vi "_CSMOFGV.vi"(6 "Operation":T3=enum."Get By Name", 7 "Allowed Messages(Empty for all)":string[](array[string]), 8 "Error in":errorcluster caption="Error in (no error)", 10 "Reference":string, 11 "Name(\"\" to use uuid) in":string) -> (0 "Error out":errorcluster, 1 "Boolean":bool, 3 "Array":T1[](array[typedef]))   [LabVIEW 2020, in "Communicable State Machine.lvlib"]
uses:
  Communicable State Machine.lvlib
  _CSMOFGVOPER.ctl
  _CSMObj.ctl
  Priority Queue.lvclass
  _CSM_MODE.ctl
  _CSMObj-Data.ctl
  _CSM Status Change Event Data.ctl
  _CSMObj-ModeData.ctl
  Def-CSMOMgr.ctl
  Priority Queue.lvclass/Priority Queue.ctl
  global-CSMQ FGV Change Flag.vi
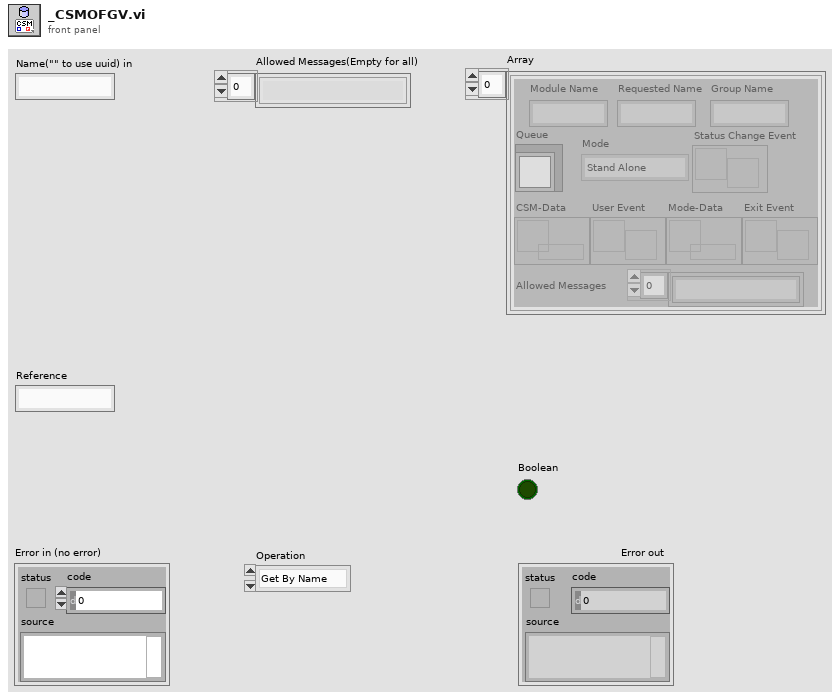
[diagram p1: front panel]
types:
  T1 = typedef "Communicable State Machine.lvlib/_CSMObj.ctl" = cluster{"Requested Name":string, "Module Name":string, "Mode":T2, "Queue":refnum<class "Priority Queue.lvclass">, "CSM-Data":refnum<data-value>, "User Event":refnum<user-event>, "Status Change Event":refnum<user-event>, "Allowed Messages":string[], "Mode-Data":refnum<data-value>, "Group Name":string, "Exit Event":refnum<user-event>}
  T2 = typedef "Communicable State Machine.lvlib/_CSM_MODE.ctl" = enum16{"Not Exist", "Stand Alone", "CSM", "Worker Agent", "Worker", "Chain", "Chain Node"}
  T3 = typedef "Communicable State Machine.lvlib/_CSMOFGVOPER.ctl" = enum16{"Create If not Exist", "Get By Name", "List", "Check If Name Exists", "Release", "Module Status", "Create Status Event Handler", "Destroy Status Event Handler"}
  T4 = typedef "Communicable State Machine.lvlib/Def-CSMOMgr.ctl" = variant
  T5 = typedef "Communicable State Machine.lvlib/_CSMObj-ModeData.ctl" = cluster{"Share Count":i32, "Messages of Chain Nodes":cluster{"Module Name":string, "Allowed Messages":string[]}[], "Chain Message Mapping Map":variant}
  T6 = cluster{"Module Name":string, "Allowed Messages":string[]}[]
  T7 = cluster{"Module Name":string, "Allowed Messages":string[]}
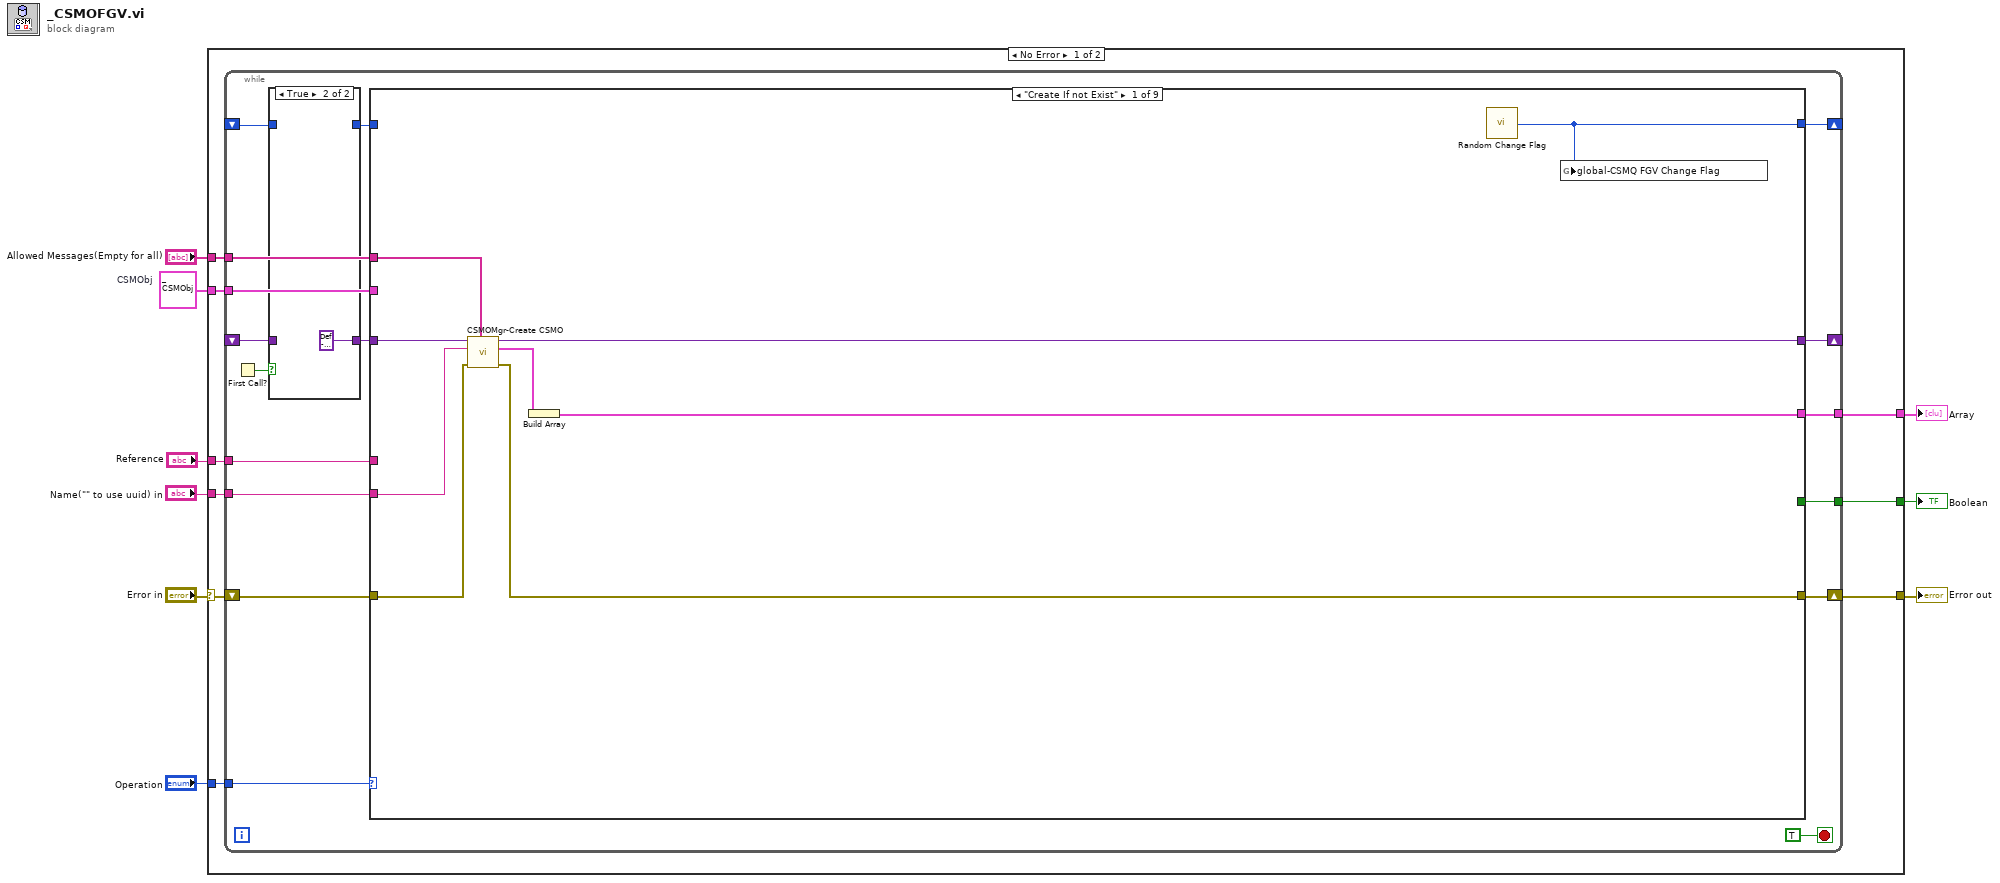
[diagram p0: block diagram]
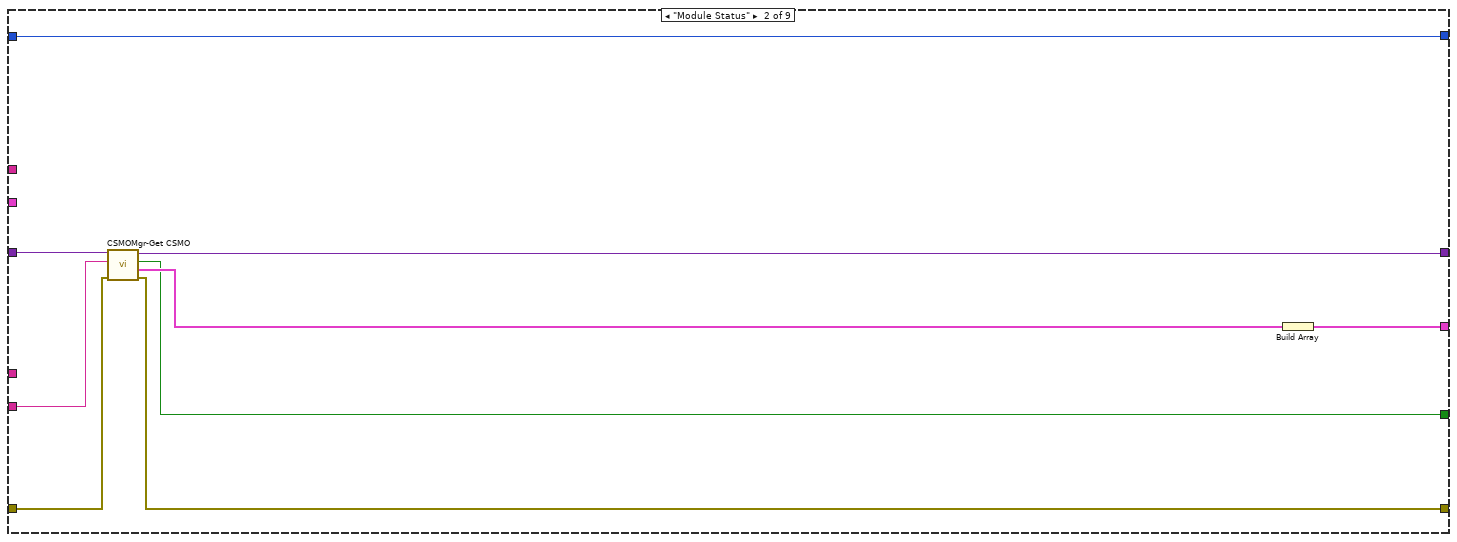
[diagram p3: hidden frame]
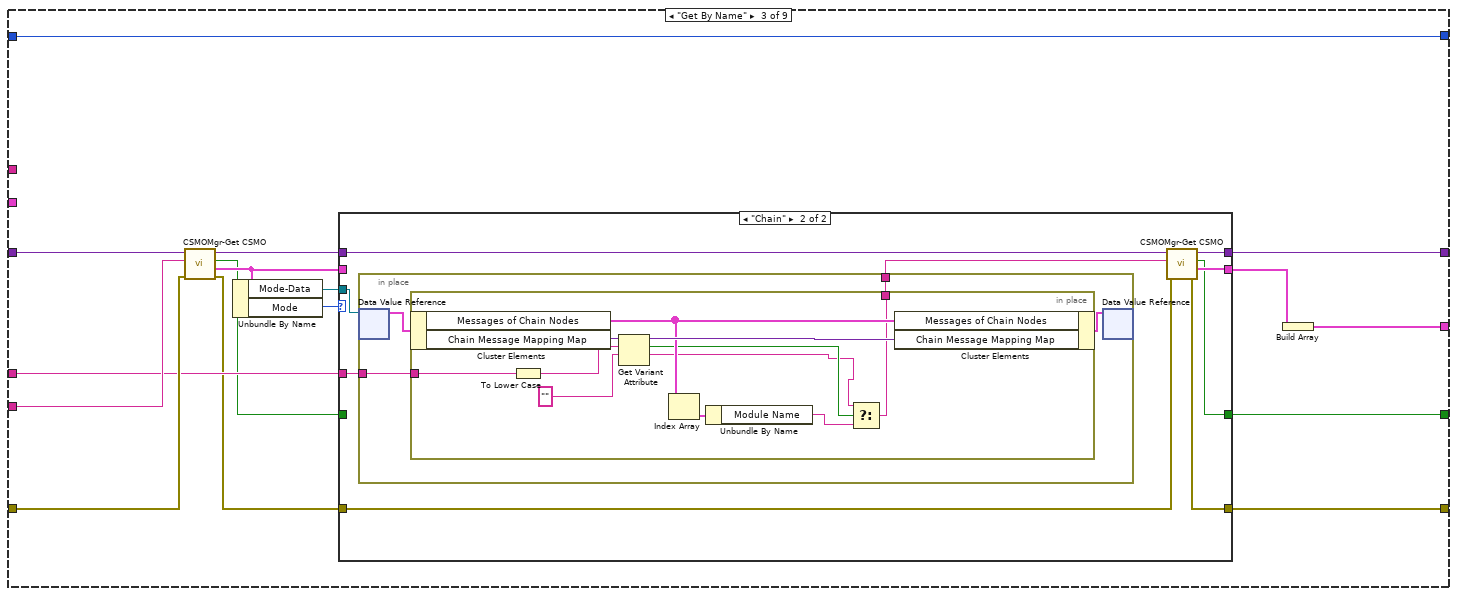
[diagram p4: hidden frame]
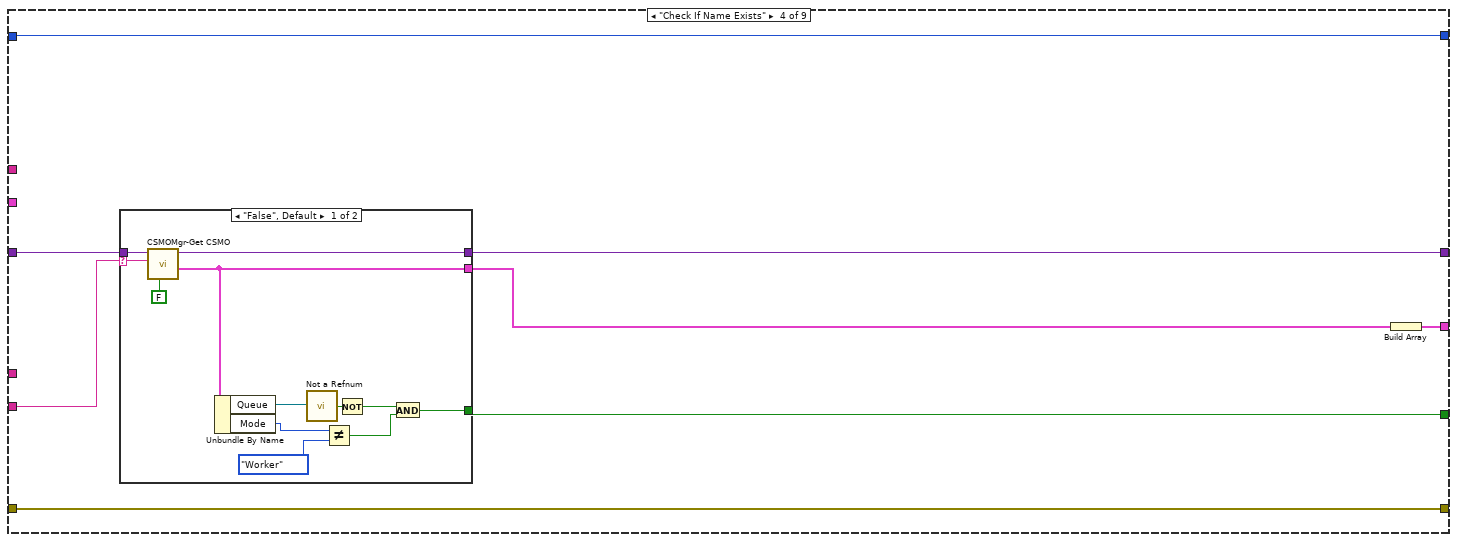
[diagram p6: hidden frame]
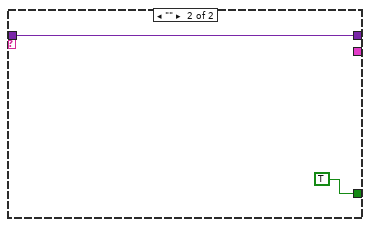
[diagram p7: hidden frame]
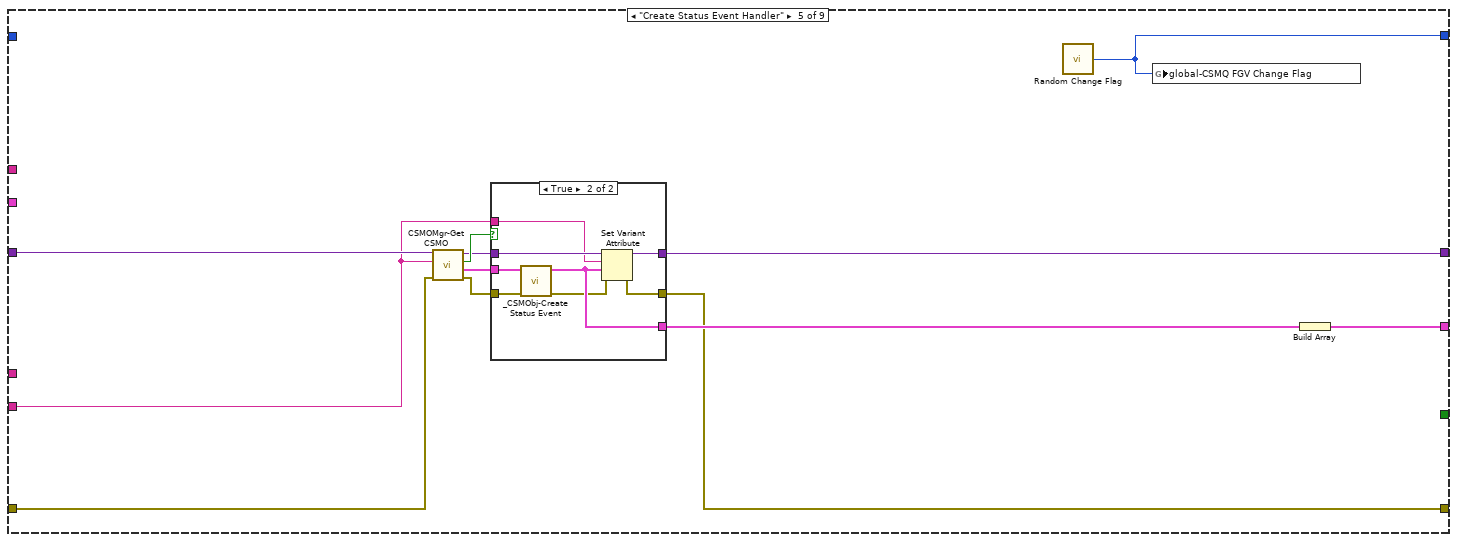
[diagram p8: hidden frame]
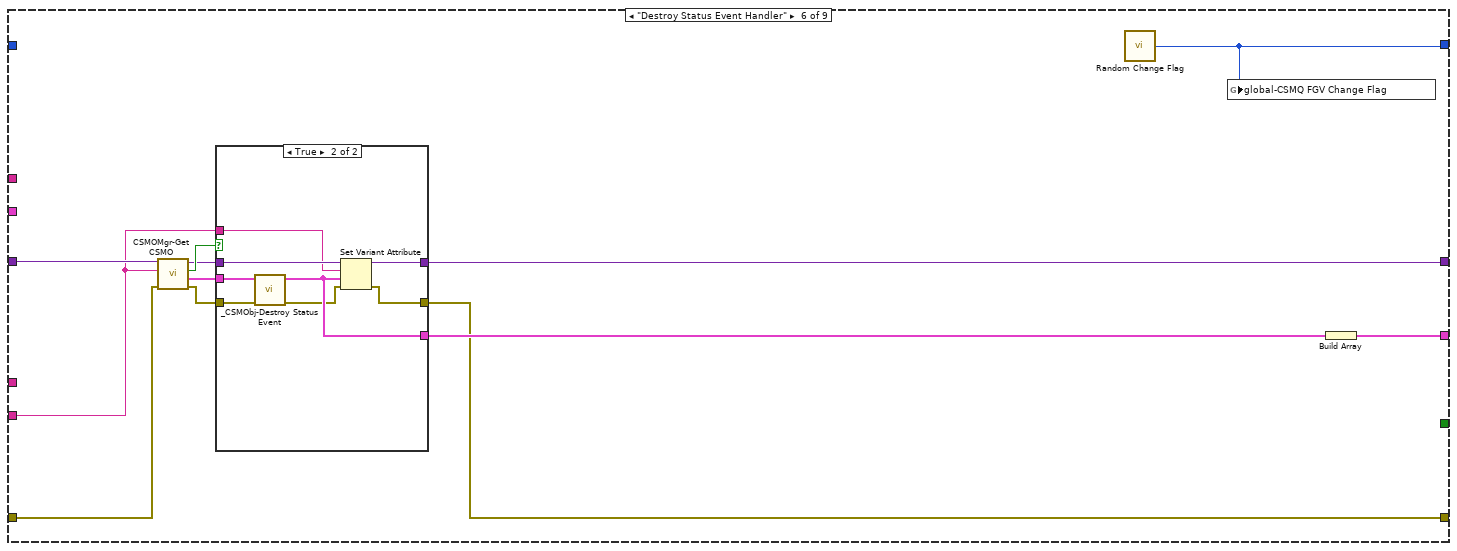
[diagram p10: hidden frame]
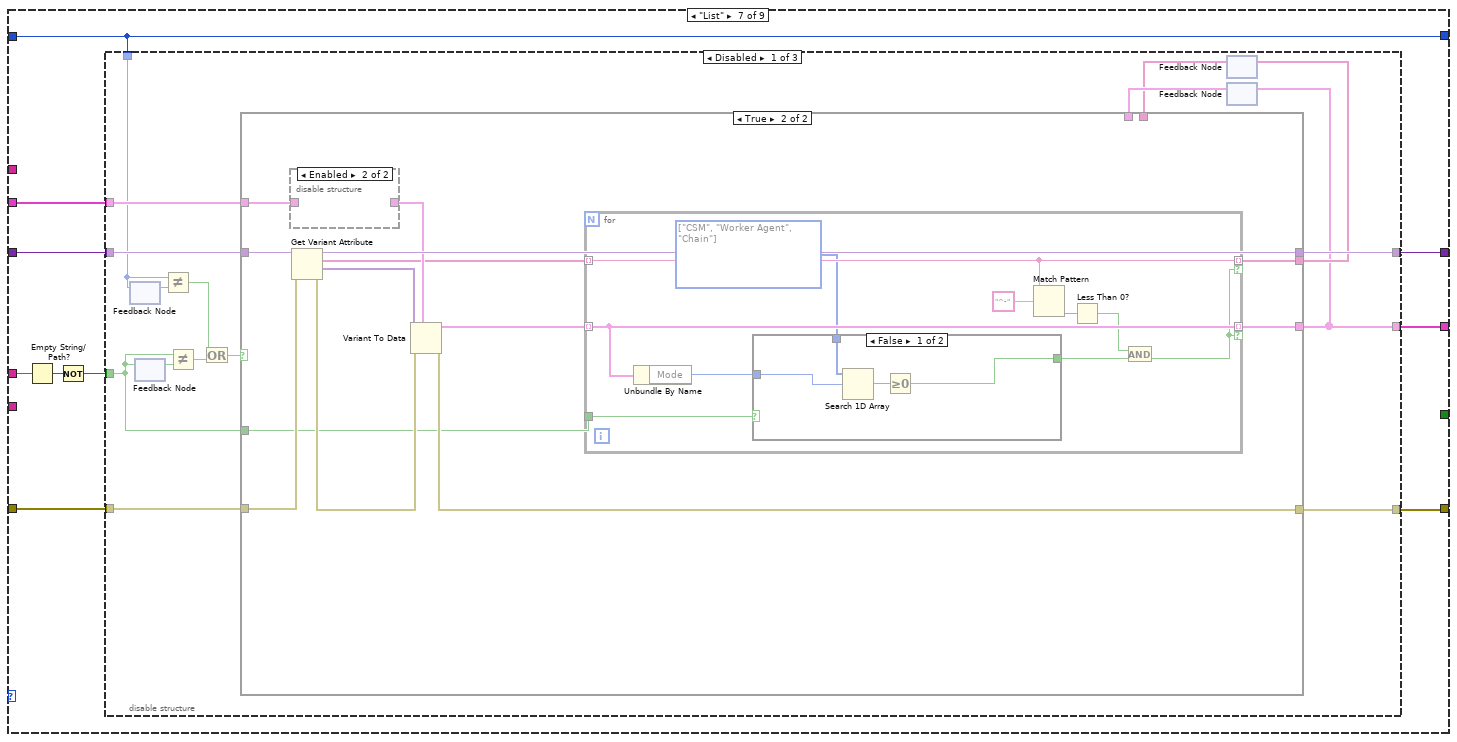
[diagram p12: hidden frame]
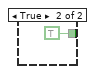
[diagram p14: hidden frame]
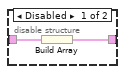
[diagram p15: hidden frame]
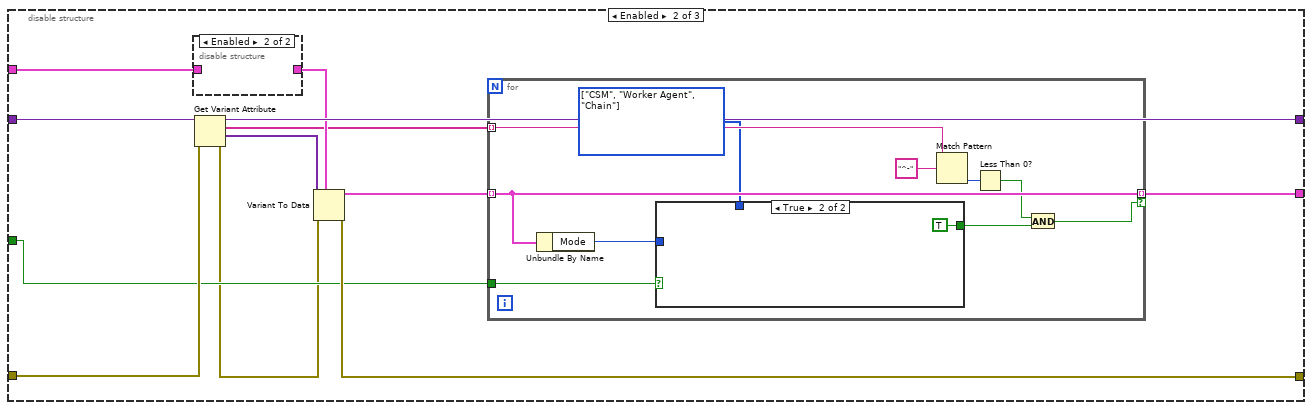
[diagram p16: hidden frame]
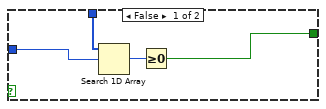
[diagram p17: hidden frame]
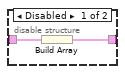
[diagram p18: hidden frame]
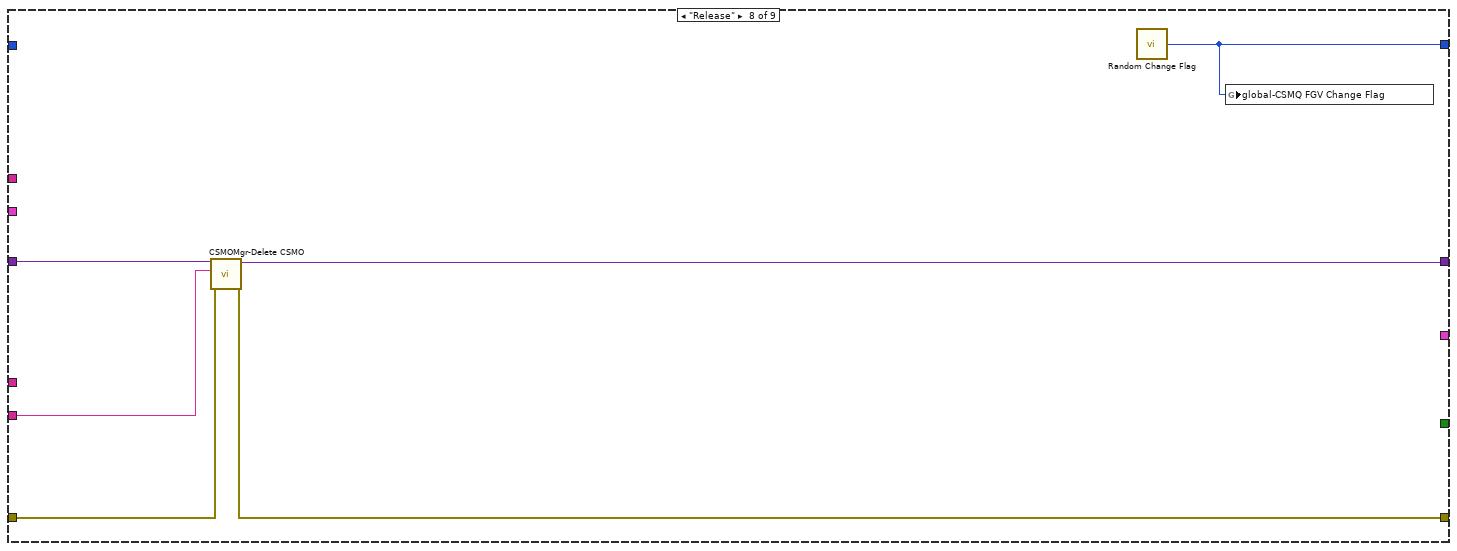
[diagram p20: hidden frame]
diagram:
  w5 = T1 {"Requested Name"="", "Module Name"="", "Mode"=enum."Stand Alone", "Queue"=refnum, "CSM-Data"=refnum, "User Event"=refnum, "Status Change Event"=refnum, "Allowed Messages"=[], "Mode-Data"=refnum, "Group Name"="", "Exit Event"=refnum}  # CSMObj
  n1 = case shown="No Error" "Error in" {
    selector: "Error in" -> [w16 w267]
    tunnel: "Operation" -> [w18 _]
    tunnel: "Name(\"\" to use uuid) in" -> [w17 _]
    tunnel: [w15 w267] -> w6
    tunnel: w5 -> [w14 _]
    tunnel: [w13 _] -> w4
    tunnel: [w12 _] -> w3
    tunnel: "Allowed Messages(Empty for all)" -> [w11 _]
    tunnel: "Reference" -> [w10 _]
    frame No Error {
      n2 = while {
        tunnel: w18 -> [w34]
        tunnel: w17 -> [w33]
        tunnel: [w32] -> w13
        shift-right: [w28] -> _
        shift-left: _ -> [w30]
        shift-right: [w26] -> w15
        shift-left: w16 -> [w27]
        tunnel: w14 -> [w25]
        tunnel: [w24] -> w12
        shift-right: [w23] -> _
        shift-left: _ -> [w21]
        tunnel: w11 -> [w20]
        tunnel: w10 -> [w19]
        stop <- TRUE stop-if-true
        n3 = First Call?() -> (First Call?: T/F=w31:bool)
        n4 = case shown="True" w31 {
          tunnel: [w37 T4 variant] -> w29
          tunnel: w30 -> [w37 _]
          tunnel: [w36 _] -> w22
          tunnel: w21 -> [w36 _]
          frame False {
          }
          frame True {
          }
        }
        n5 = case shown="\"Create If not Exist\"" w34 {
          tunnel: w33 -> [w40 w48 w68 w101 w133 w156 _ w261 _]
          tunnel: [w43 w53 w71 w105 w127 w150 w172 _ _] -> w32
          tunnel: w29 -> [w41 w56 w72 w102 w134 w157 w178 w263 w266]
          tunnel: [w47 w55 w64 w108 w129 w152 w177 w260 w266] -> w28
          tunnel: w27 -> [w44 w51 w69 w106 w126 w149 w175 w262 w265]
          tunnel: [w46 w50 w57 w106 w124 w147 w174 w259 w265] -> w26
          tunnel: w25 -> [_ _ _ _ _ _ w176 _ _]
          tunnel: [_ w49 w58 w104 _ _ _ _ _] -> w24
          tunnel: w22 -> [_ w52 w70 w103 _ _ w173 _ w264]
          tunnel: [w39 w52 w70 w103 w123 w146 w173 w258 w264] -> w23
          tunnel: w20 -> [w42 _ _ _ _ _ _ _ _]
          tunnel: w19 -> [_ _ w62 _ _ _ w170 _ _]
          frame "Create If not Exist" {
            n6 = call "CSMOMgr-Create CSMO.vi"("Allowed Messages(Empty for all)"=w42, "error in (no error)"=w44, "Name(\"\" to use uuid) in"=w40, "CSMOMgr"=w41) -> ("error out"=w46:errorcluster, "CSMO"=w45:T1, "CSMOMgr out"=w47:T4)  [unwired: 5 in]
            n7 = Build Array(w45) -> (w43:T1[])
            n8 = call "Random Change Flag.vi"() -> ("Random Change Flag"=w39:u64)  [unwired: 2 in]
            n9 = global write "global-CSMQ FGV Change Flag.vi" "global-CSMQ FGV Change Flag"(w39) -> ()
          }
          frame "Module Status" {
            n10 = call "CSMOMgr-Get CSMO.vi"("Error in"=w51, "Queue Name"=w48, "CSMOMgr"=w56) -> ("Error out"=w50:errorcluster, "values"=w54:T1, "found"=w49:bool, "CSMOMgr out"=w55:T4)  [unwired: 5 in]
            n11 = Build Array(w54) -> (w53:T1[])
          }
          frame "Get By Name" {
            n12 = call "CSMOMgr-Get CSMO.vi"("Error in"=w69, "Queue Name"=w68, "CSMOMgr"=w72) -> ("Error out"=w60:errorcluster, "values"=w66:T1, "found"=w59:bool, "CSMOMgr out"=w63:T4)  [unwired: 5 in]
            n13 = Unbundle By Name(w66) -> ("Mode-Data"=w61:refnum<data-value>, "Mode"=w67:T2)
            n14 = case shown="\"Chain\"" w67 {
              tunnel: w66 -> [w76 _]
              tunnel: [w76 w83] -> w65
              tunnel: [w75 w78] -> w64
              tunnel: w63 -> [w75 w79]
              tunnel: w62 -> [_ w84]
              tunnel: w61 -> [_ w85]
              tunnel: w60 -> [w73 w81]
              tunnel: w59 -> [w74 _]
              tunnel: [w74 w82] -> w58
              tunnel: [w73 w80] -> w57
              frame "Not Exist", Default {
              }
              frame "Chain" {
                n15 = in-place {
                  in-place-border: w84 -> [w87]
                  in-place-border: [w86] -> w77
                  n16 = in-place-dvr #1(w85) -> (w89:T5)  [unwired: 1 out]
                  n17 = in-place {
                    in-place-border: w87 -> [w98]
                    in-place-border: [w92] -> w86
                    n18 = in-place-cluster #2(w89) -> ("Messages of Chain Nodes"=w95:T6, "Chain Message Mapping Map"=w100:variant)
                    n19 = To Lower Case(string=w98) -> (all lower case string=w96:string)
                    n20 = Get Variant Attribute(Variant=w100, name=w96, default value (empty Variant)="") -> (duplicate Variant=w99:variant, found=w93:bool, value=w91:string)  [unwired: 1 in, 1 out]
                    n21 = Index Array(array=w95) -> (element=w94:T7)  [unwired: 1 in]
                    n22 = Unbundle By Name(w94) -> ("Module Name"=w90:string)
                    n23 = Select(t=w91, s=w93, f=w90) -> (s? t:f=w92:string)
                    n24 = in-place-cluster #2("Messages of Chain Nodes"=w95, "Chain Message Mapping Map"=w99) -> (w88:T5)
                  }
                  n25 = in-place-dvr #1(w88) -> ()  [unwired: 2 out]
                }
                n26 = call "CSMOMgr-Get CSMO.vi"("Error in"=w81, "Queue Name"=w77, "CSMOMgr"=w79) -> ("Error out"=w80:errorcluster, "values"=w83:T1, "found"=w82:bool, "CSMOMgr out"=w78:T4)  [unwired: 5 in]
              }
            }
            n27 = Build Array(w65) -> (w71:T1[])
          }
          frame "Check If Name Exists" {
            n28 = case shown="\"False\", Default" w101 {
              selector: w101 -> [w111 _]
              tunnel: w102 -> [w113 w122]
              tunnel: [w112 w122] -> w108
              tunnel: [w110 _] -> w107
              tunnel: [w117 TRUE] -> w104
              frame "False", Default {
                n29 = call "CSMOMgr-Get CSMO.vi"("GenError?(T)"=FALSE, "Queue Name"=w111, "CSMOMgr"=w113) -> ("values"=w110:T1, "CSMOMgr out"=w112:T4)  [unwired: 5 in, 2 out]
                n30 = Unbundle By Name(w110) -> ("Queue"=w120:refnum<class "Priority Queue.lvclass">, "Mode"=w116:T2)
                n31 = call "Not a Refnum.vi"("Priority Queue.lvclass"=w120) -> ("NaN/Path/Refnum?"=w119:bool)  [unwired: 4 in]
                n32 = Not Equal?(x=w116, y=_CSM_MODE."Worker") -> (x != y?=w114:bool)
                n33 = Not(x=w119) -> (.not. x?=w118:bool)
                n34 = And(x=w118, y=w114) -> (x .and. y?=w117:bool)
              }
              frame "" {
              }
            }
            n35 = Build Array(w107) -> (w105:T1[])
          }
          frame "Create Status Event Handler" {
            n36 = call "CSMOMgr-Get CSMO.vi"("Error in"=w126, "Queue Name"=w133, "CSMOMgr"=w134) -> ("Error out"=w125:errorcluster, "values"=w132:T1, "found"=w131:bool, "CSMOMgr out"=w130:T4)  [unwired: 5 in]
            n37 = case shown="True" w131 {
              tunnel: w132 -> [w136 w142]
              tunnel: w130 -> [w137 w145]
              tunnel: [w137 w144] -> w129
              tunnel: w133 -> [_ w143]
              tunnel: [w136 w141] -> w128
              tunnel: w125 -> [w135 w140]
              tunnel: [w135 w138] -> w124
              frame False {
              }
              frame True {
                n38 = call "_CSMObj-Create Status Event.vi"("Error in"=w140, "values in"=w142) -> ("Error out"=w139:errorcluster, "values out"=w141:T1)  [unwired: 8 in]
                n39 = Set Variant Attribute(Variant=w145, name=w143, value=w141, error in=w139) -> (Variant out=w144:T4, error out=w138:errorcluster)  [unwired: 1 out]
              }
            }
            n40 = call "Random Change Flag.vi"() -> ("Random Change Flag"=w123:u64)  [unwired: 2 in]
            n41 = global write "global-CSMQ FGV Change Flag.vi" "global-CSMQ FGV Change Flag"(w123) -> ()
            n42 = Build Array(w128) -> (w127:T1[])
          }
          frame "Destroy Status Event Handler" {
            n43 = call "CSMOMgr-Get CSMO.vi"("Error in"=w149, "Queue Name"=w156, "CSMOMgr"=w157) -> ("Error out"=w148:errorcluster, "values"=w155:T1, "found"=w154:bool, "CSMOMgr out"=w153:T4)  [unwired: 5 in]
            n44 = case shown="True" w154 {
              tunnel: w155 -> [w159 w165]
              tunnel: w153 -> [w160 w168]
              tunnel: [w160 w167] -> w152
              tunnel: w156 -> [_ w166]
              tunnel: [w159 w164] -> w151
              tunnel: w148 -> [w158 w163]
              tunnel: [w158 w161] -> w147
              frame False {
              }
              frame True {
                n45 = call "_CSMObj-Destroy Status Event.vi"("Error in"=w163, "values in"=w165) -> ("Error out"=w162:errorcluster, "values out"=w164:T1)  [unwired: 8 in]
                n46 = Set Variant Attribute(Variant=w168, name=w166, value=w164, error in=w162) -> (Variant out=w167:T4, error out=w161:errorcluster)  [unwired: 1 out]
              }
            }
            n47 = call "Random Change Flag.vi"() -> ("Random Change Flag"=w146:u64)  [unwired: 2 in]
            n48 = global write "global-CSMQ FGV Change Flag.vi" "global-CSMQ FGV Change Flag"(w146) -> ()
            n49 = Build Array(w151) -> (w150:T1[])
          }
          frame "List" {
            n50 = Empty String/Path?(string/path=w170) -> (empty?=w171:bool)
            n51 = Not(x=w171) -> (.not. x?=w169:bool)
            n52 = disable-structure shown="Disabled" {
              disable-tunnel: w178 -> [w194 w240 _]
              disable-tunnel: [w193 w239 _] -> w177
              disable-tunnel: w176 -> [w192 w238 _]
              disable-tunnel: w175 -> [w191 w237 _]
              disable-tunnel: [w190 w236 _] -> w174
              disable-tunnel: w173 -> [w188 _ _]
              disable-tunnel: [w182 w235 _] -> w172
              disable-tunnel: w169 -> [w179 w234 _]
              frame Disabled {
                n53 = feedback #3() -> (w189:u64)  [unwired: 1 in]
                n54 = feedback-in #3(w188) -> ()
                n55 = feedback #4() -> (w187:bool)  [unwired: 1 in]
                n56 = feedback-in #4(w179) -> ()
                n57 = Not Equal?(x=w188, y=w189) -> (x != y?=w185:bool)
                n58 = Not Equal?(x=w179, y=w187) -> (x != y?=w186:bool)
                n59 = Or(x=w185, y=w186) -> (x .or. y?=w184:bool)
                n60 = feedback #5() -> (w180:string[])  [unwired: 1 in]
                n61 = feedback #6() -> (w181:T1[])  [unwired: 1 in]
                n62 = case shown="True" w184 {
                  tunnel: w194 -> [w196 w211]
                  tunnel: [w196 w210] -> w193
                  tunnel: w192 -> [_ w208]
                  tunnel: [w197 w204] -> w183
                  tunnel: [w198 w203] -> w182
                  tunnel: w191 -> [w195 w201]
                  tunnel: [w195 w200] -> w190
                  tunnel: w179 -> [_ w199]
                  tunnel: w181 -> [w198 _]
                  tunnel: w180 -> [w197 _]
                  frame False {
                  }
                  frame True {
                    n63 = disable-structure shown="Enabled" {
                      disable-tunnel: w208 -> [w228 _]
                      disable-tunnel: [w227 _] -> w207
                      frame Disabled {
                        n64 = Build Array(w228) -> (w227:T1[])
                      }
                      frame Enabled {
                      }
                    }
                    n65 = Get Variant Attribute(Variant=w211, error in=w201) -> (duplicate Variant=w210:variant, names=w205:string[], values=w209:variant[], error out=w202:errorcluster)  [unwired: 2 in]
                    n66 = Variant To Data(error in=w202, type=w207, Variant=w209) -> (data=w206:T1[], error out=w200:errorcluster)
                    n67 = for {
                      tunnel: w206 -> [w221] mode=indexing
                      tunnel: w205 -> [w216] mode=indexing
                      tunnel: [w216] -> w204 mode=indexing if=w217
                      tunnel: [w221] -> w203 mode=indexing if=w217
                      tunnel: w199 -> [w218]
                      w212 = T2[] [enum."CSM", enum."Worker Agent", enum."Chain"] items=["Not Exist", "Stand Alone", "CSM", "Worker Agent", "Worker", "Chain", "Chain Node"]
                      n68 = Unbundle By Name(w221) -> ("Mode"=w220:T2)
                      n69 = case shown="False" w218 {
                        tunnel: [w222 TRUE] -> w219
                        tunnel: w220 -> [w225 _]
                        tunnel: w212 -> [w224 _]
                        frame False {
                          n70 = Search 1D Array(1D array=w224, element=w225) -> (index of element=w223:i32)  [unwired: 1 in]
                          n71 = Greater Or Equal To 0?(x=w223) -> (x >= 0?=w222:bool)
                        }
                        frame True {
                        }
                      }
                      n72 = Match Pattern(string=w216, regular expression="^-") -> (offset past match=w214:i32)  [unwired: 1 in, 3 out]
                      n73 = Less Than 0?(x=w214) -> (x < 0?=w213:bool)
                      n74 = And(x=w213, y=w219) -> (x .and. y?=w217:bool)
                    }
                  }
                }
                n75 = feedback-in #5(w183) -> ()
                n76 = feedback-in #6(w182) -> ()
              }
              frame Enabled {
                n77 = disable-structure shown="Enabled" {
                  disable-tunnel: w238 -> [w257 _]
                  disable-tunnel: [w256 _] -> w232
                  frame Disabled {
                    n78 = Build Array(w257) -> (w256:T1[])
                  }
                  frame Enabled {
                  }
                }
                n79 = Get Variant Attribute(Variant=w240, error in=w237) -> (duplicate Variant=w239:variant, names=w230:string[], values=w233:variant[], error out=w229:errorcluster)  [unwired: 2 in]
                n80 = Variant To Data(error in=w229, type=w232, Variant=w233) -> (data=w231:T1[], error out=w236:errorcluster)
                n81 = for {
                  tunnel: w231 -> [w250] mode=indexing
                  tunnel: w230 -> [w245] mode=indexing
                  tunnel: [w250] -> w235 mode=indexing if=w246
                  tunnel: w234 -> [w247]
                  w241 = T2[] [enum."CSM", enum."Worker Agent", enum."Chain"] items=["Not Exist", "Stand Alone", "CSM", "Worker Agent", "Worker", "Chain", "Chain Node"]
                  n82 = Unbundle By Name(w250) -> ("Mode"=w249:T2)
                  n83 = case shown="True" w247 {
                    tunnel: [w251 TRUE] -> w248
                    tunnel: w249 -> [w254 _]
                    tunnel: w241 -> [w253 _]
                    frame False {
                      n84 = Search 1D Array(1D array=w253, element=w254) -> (index of element=w252:i32)  [unwired: 1 in]
                      n85 = Greater Or Equal To 0?(x=w252) -> (x >= 0?=w251:bool)
                    }
                    frame True {
                    }
                  }
                  n86 = Match Pattern(string=w245, regular expression="^-") -> (offset past match=w243:i32)  [unwired: 1 in, 3 out]
                  n87 = Less Than 0?(x=w243) -> (x < 0?=w242:bool)
                  n88 = And(x=w242, y=w248) -> (x .and. y?=w246:bool)
                }
              }
              frame Disabled {
              }
            }
          }
          frame "Release" {
            n89 = call "CSMOMgr-Delete CSMO.vi"("Error in"=w262, "Queue Name"=w261, "CSMOMgr"=w263) -> ("Error out"=w259:errorcluster, "CSMOMgr out"=w260:T4)  [unwired: 7 in]
            n90 = call "Random Change Flag.vi"() -> ("Random Change Flag"=w258:u64)  [unwired: 2 in]
            n91 = global write "global-CSMQ FGV Change Flag.vi" "global-CSMQ FGV Change Flag"(w258) -> ()
          }
          frame Default {
          }
        }
      }
    }
    frame Error {
    }
  }
  "Error out" <- w6
  "Array" <- w4
  "Boolean" <- w3
